vi "11 DAQ Config (continuous) (2017).vi"(0 "Error In":errorcluster) -> (1 "task out":refnum<k21>, 2 "Error Out":errorcluster)   [LabVIEW 2017]
uses:
  <vilib>/DAQmx/create/channels.llb/DAQmx Create Channel (AI-Voltage-Basic).vi
  <vilib>/DAQmx/configure/timing.llb/DAQmx Timing (Sample Clock).vi
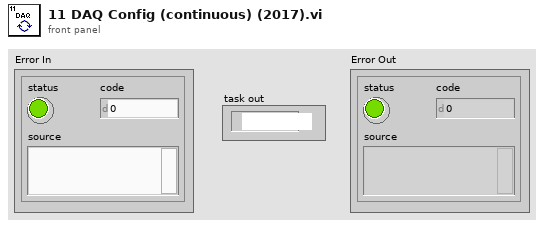
[diagram p1: front panel]
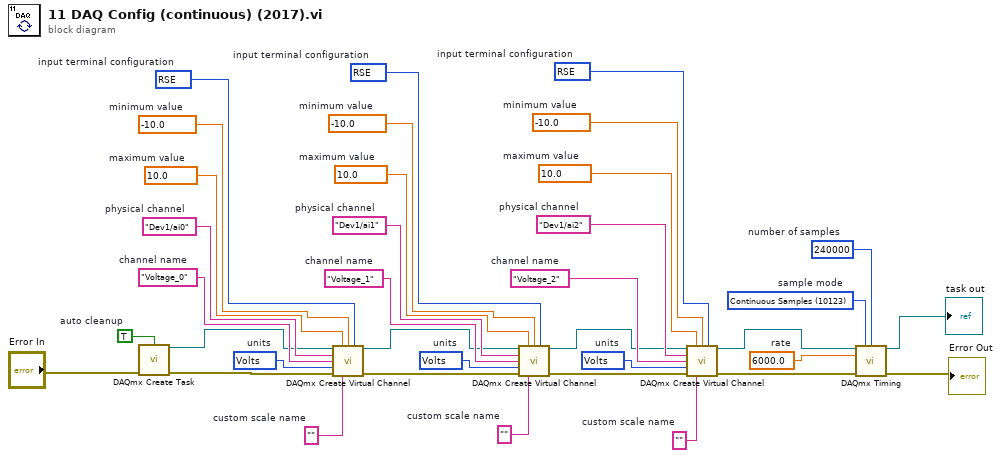
[diagram p0: block diagram]
diagram:
  w35 = 10123 items=["Finite Samples"=10178, "Continuous Samples"=10123, "Hardware Timed Single Point"=12522]  # sample mode
  w34 = 240000  # number of samples
  w33 = 6000.0  # rate
  w31 = 10083 items=["default"=-1, "RSE"=10083, "NRSE"=10078, "Differential"=10106, "Pseudodifferential"=12529]  # input terminal configuration
  w30 = 10348 items=["Volts"=10348, "From Custom Scale"=10065]  # units
  w29 = "Voltage_2"  # channel name
  w27 = ""  # custom scale name
  w26 = -10.0  # minimum value
  w25 = 10.0  # maximum value
  w24 = "Dev1/ai2"  # physical channel
  w22 = 10083 items=["default"=-1, "RSE"=10083, "NRSE"=10078, "Differential"=10106, "Pseudodifferential"=12529]  # input terminal configuration
  w21 = 10348 items=["Volts"=10348, "From Custom Scale"=10065]  # units
  w20 = "Voltage_1"  # channel name
  w18 = ""  # custom scale name
  w17 = -10.0  # minimum value
  w16 = 10.0  # maximum value
  w15 = "Dev1/ai1"  # physical channel
  w13 = 10083 items=["default"=-1, "RSE"=10083, "NRSE"=10078, "Differential"=10106, "Pseudodifferential"=12529]  # input terminal configuration
  w12 = 10348 items=["Volts"=10348, "From Custom Scale"=10065]  # units
  w11 = "Voltage_0"  # channel name
  w9 = ""  # custom scale name
  w8 = -10.0  # minimum value
  w7 = 10.0  # maximum value
  w6 = "Dev1/ai0"  # physical channel
  w4 = TRUE  # auto cleanup
  n1 = call <vilib>:"DAQmx Create Task.vi"("auto cleanup"=w4, "error in"="Error In") -> ("task out"=w5:refnum<k21>, "error out"=w3:errorcluster)  [unwired: 12 in]
  n2 = call-poly <vilib>:"DAQmx Create Virtual Channel.vi"("task in"=w5, "maximum value"=w7, "minimum value"=w8, "input terminal configuration"=w13, "physical channels"=w6, "name to assign"=w11, "units"=w12, "error in"=w3, "custom scale name"=w9) -> ("task out"=w14:refnum<k21>, "error out"=w10:errorcluster)  [unwired: 5 in]
  n3 = call-poly <vilib>:"DAQmx Create Virtual Channel.vi"("task in"=w14, "maximum value"=w16, "minimum value"=w17, "input terminal configuration"=w22, "physical channels"=w15, "name to assign"=w20, "units"=w21, "error in"=w10, "custom scale name"=w18) -> ("task out"=w23:refnum<k21>, "error out"=w19:errorcluster)  [unwired: 5 in]
  n4 = call-poly <vilib>:"DAQmx Create Virtual Channel.vi"("task in"=w23, "maximum value"=w25, "minimum value"=w26, "input terminal configuration"=w31, "physical channels"=w24, "name to assign"=w29, "units"=w30, "error in"=w19, "custom scale name"=w27) -> ("task out"=w32:refnum<k21>, "error out"=w28:errorcluster)  [unwired: 5 in]
  n5 = call-poly <vilib>:"DAQmx Timing.vi"("task/channels in"=w32, "sample mode"=w35, "samples per channel"=w34, "rate"=w33, "error in"=w28) -> ("task out"=→"task out":refnum<k21>, "error out"=→"Error Out":errorcluster)  [unwired: 9 in]
